vi "Configure Deviation Measurement.vi"(5 "Reference Value B (0.0)":dbl, 7 "Deviation Mode B (0: Off)":u16(ring) items=["Off", "Absolute", "Percent"], 8 "error in (no error)":errorcluster, 9 "Reference Value A (0.0)":dbl, 10 "Deviation Mode A (0: Off)":u16(ring) items=["Off", "Absolute", "Percent"], 11 "VISA resource name":refnum<visa-resource-name>) -> (0 "error out":errorcluster, 3 "VISA resource name out":refnum<visa-resource-name>)   [LabVIEW 2017, in "Agilent E4980.lvlib"]
doc: "Sets the deviation mode as well as the deviation reference for both primary and secondary parameters.\n\n<B>Notes:</B>\n(1) The deviation measurement feature allows you to display deviation values instead of actual measurements. A deviation is expressed as the difference between the actual measurement and the stored reference value. \n\n(2) The deviation measurement feature is useful when you observe how the measurement results change under varying conditions of temperature, frequency, bias, and other influences."
uses:
  Agilent E4980.lvlib
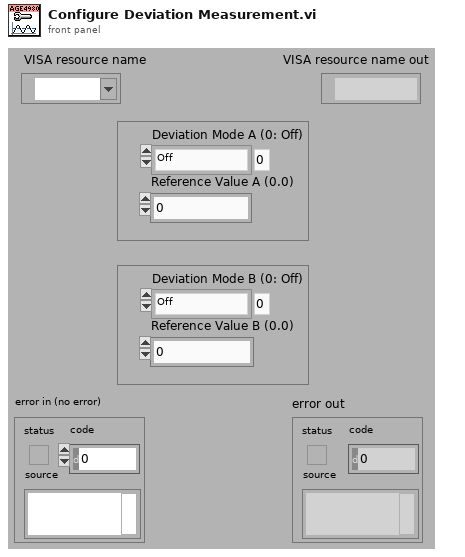
[diagram p1: front panel]
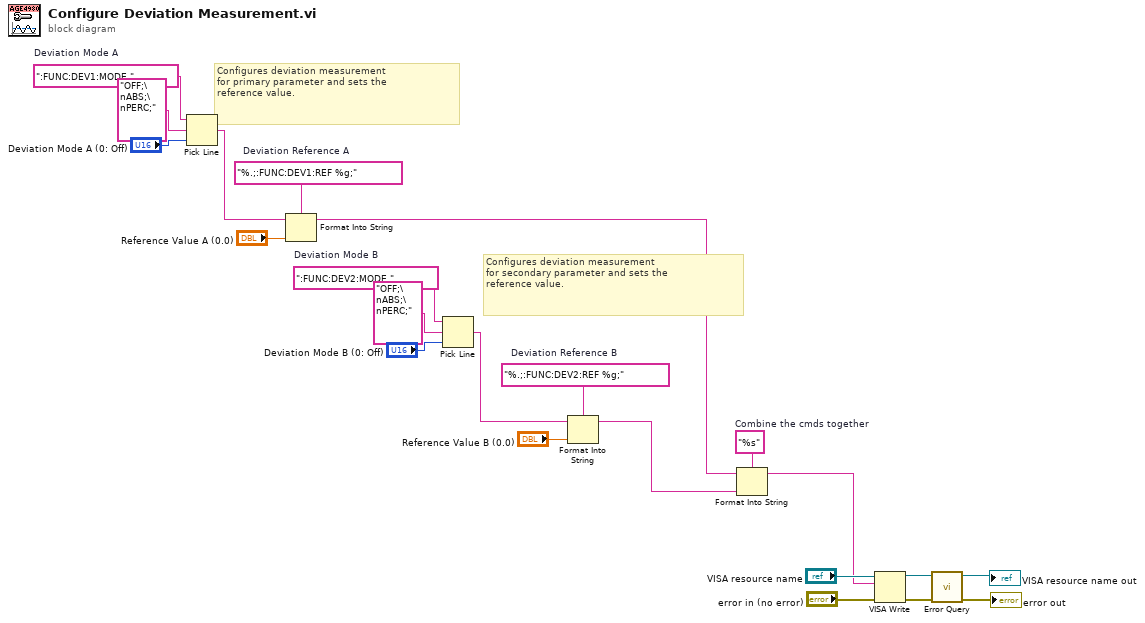
[diagram p0: block diagram]
diagram:
  w12 = "%s"  # Combine the cmds together
  w14 = "%.;:FUNC:DEV2:REF %g;"  # Deviation Reference B
  w16 = ":FUNC:DEV2:MODE "  # Deviation Mode B
  w18 = "%.;:FUNC:DEV1:REF %g;"  # Deviation Reference A
  w20 = ":FUNC:DEV1:MODE "  # Deviation Mode A
  # "Configures deviation measurement\nfor secondary parameter and sets the\nreference value."
  # "Configures deviation measurement\nfor primary parameter and sets the\nreference value."
  n1 = Pick Line(string ("")=w20, multi-line string="OFF;\nABS;\nPERC;", line index="Deviation Mode A (0: Off)") -> (output string=w19:string)
  n2 = Format Into String(format string=w18, initial string=w19, "Reference Value A (0.0)") -> (resulting string=w2:string)  [unwired: 1 in, 1 out]
  n3 = Pick Line(string ("")=w16, multi-line string="OFF;\nABS;\nPERC;", line index="Deviation Mode B (0: Off)") -> (output string=w15:string)
  n4 = Format Into String(format string=w14, initial string=w15, "Reference Value B (0.0)") -> (resulting string=w1:string)  [unwired: 1 in, 1 out]
  n5 = Format Into String(format string=w12, initial string=w2, w1) -> (resulting string=w9:string)  [unwired: 1 in, 1 out]
  n6 = VISA Write(VISA resource name="VISA resource name", write buffer=w9, error in (no error)="error in (no error)") -> (VISA resource name out=w8:refnum<visa-resource-name>, error out=w7:errorcluster)  [unwired: 1 out]
  n7 = call "Error Query.vi"("error in (no error)"=w7, "VISA resource name"=w8) -> ("error out"=→"error out":errorcluster, "VISA resource name out"=→"VISA resource name out":refnum<visa-resource-name>)  [unwired: 6 in, 2 out]
